vi "daq_FSM.vi"(8 "loop rate":u32=1000, 9 "commands":refnum<queue>, 11 "measurements":refnum<queue>) -> ()   [LabVIEW 2021, in "DAQ.lvlib"]
uses:
  DAQ.lvlib
  <vilib>/DAQmx/read.llb/DAQmx Read (Analog 1D DBL 1Chan NSamp).vi
  <vilib>/Analysis/baseanly.llb/Mean (DBL).vi
  <vilib>/DAQmx/create/channels.llb/DAQmx Create Channel (AI-Voltage-Basic).vi
  <vilib>/DAQmx/configure/timing.llb/DAQmx Timing (Sample Clock).vi
  <vilib>/DAQmx/miscellaneous.llb/DAQmx Fill In Error Info.vi
  <vilib>/Analysis/NI_AALBase.lvlib
panel:
  in  "STOP":bool
  out "Waveform Graph":dbl[](graph)
  in  "rate":dbl=1000.0 format="%0.2f"
  in  "samples per channel":i32=1000
  in  "physical channels":tag="Dev1/ai0"
  in  "error in":errorcluster
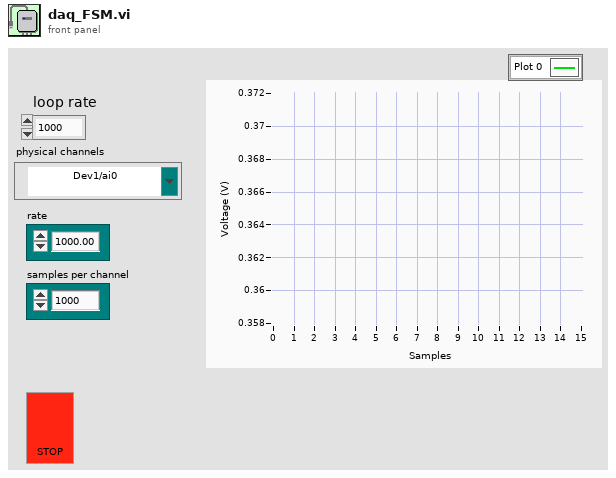
[diagram p1: front panel]
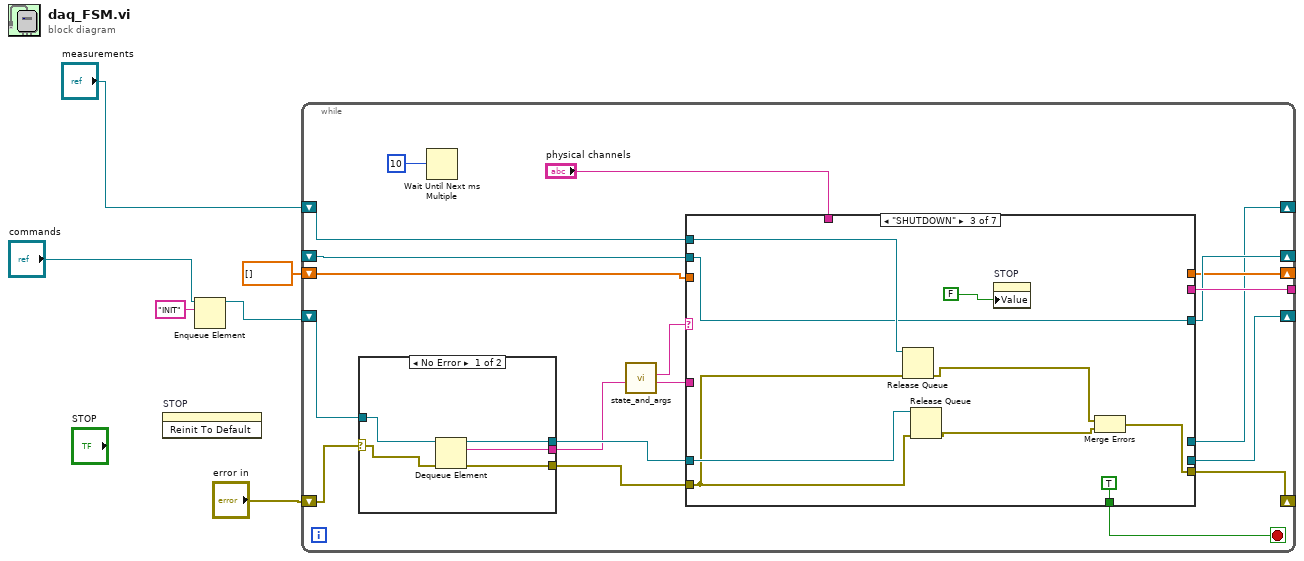
[diagram p0: block diagram]
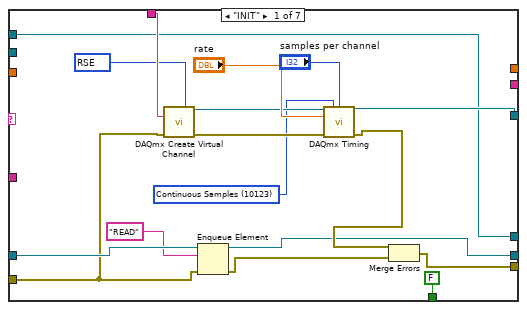
[diagram p2: hidden frame]
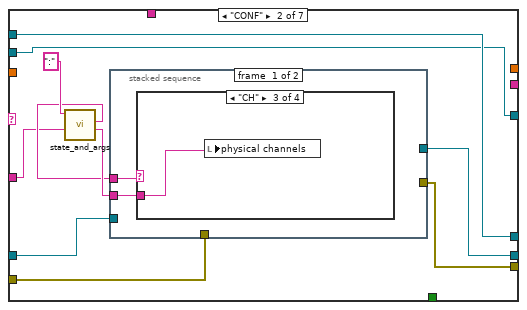
[diagram p3: hidden frame]
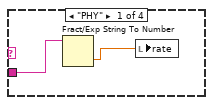
[diagram p4: hidden frame]
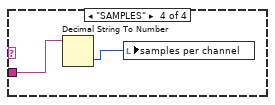
[diagram p6: hidden frame]
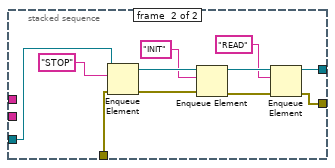
[diagram p7: hidden frame]
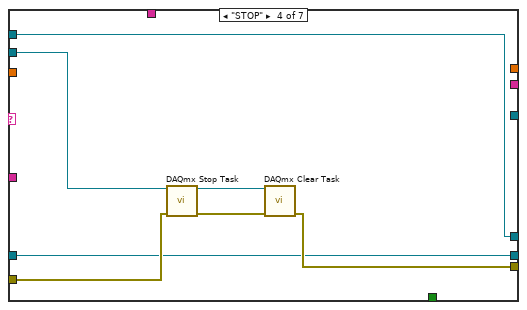
[diagram p8: hidden frame]
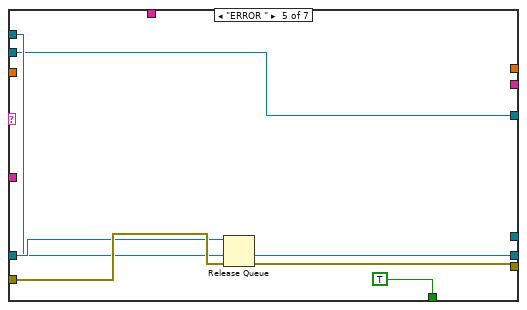
[diagram p9: hidden frame]
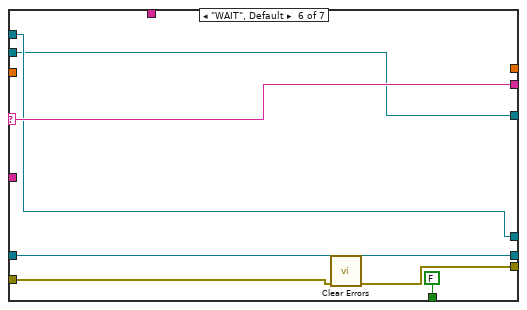
[diagram p10: hidden frame]
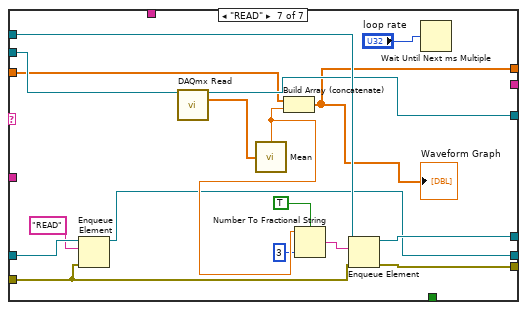
[diagram p11: hidden frame]
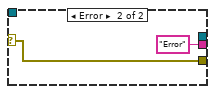
[diagram p12: hidden frame]
diagram:
  n1 = invoke on="STOP" class="Bool" method="Reinit To Default"() -> ()  [unwired: 3 in, 3 out]
  n2 = Enqueue Element(queue="commands", element="INIT") -> (queue out=w4:refnum<queue>)  [unwired: 2 in, 2 out]
  n3 = while {
    shift-right: [w15] -> _
    shift-left: "error in" -> [w25]
    tunnel: [w23] -> _
    shift-right: [w20] -> _
    shift-left: _ -> [w18]
    shift-right: [w10] -> _
    shift-left: dbl[] [] -> [w11]
    shift-right: [w8] -> _
    shift-left: w4 -> [w22]
    shift-right: [w9] -> _
    shift-left: "measurements" -> [w17]
    stop <- w14 stop-if-true
    n4 = case shown="No Error" w25 {
      selector: w25 -> [w119 w122]
      tunnel: [w121 "Error"] -> w13
      tunnel: w22 -> [w120 _]
      tunnel: [w118 w122] -> w21
      tunnel: [w117 _] -> w16
      frame No Error {
        n5 = Dequeue Element(queue=w120, error in (no error)=w119) -> (queue out=w117:refnum<queue>, element=w121:string, error out=w118:errorcluster)  [unwired: 1 in, 1 out]
      }
      frame Error {
      }
    }
    n6 = Wait Until Next ms Multiple(millisecond multiple=u32 10 ("millisecond timer value")) -> ()  [unwired: 1 out]
    n7 = call "state_and_args.vi"("String"=w13) -> ("Arguments"=w7:string, "State"=w12:string)  [unwired: 9 in]
    n8 = case shown="\"SHUTDOWN\"" w12 {
      selector: w12 -> [_ _ _ _ _ w99 _]
      tunnel: [_ _ _ _ _ w99 _] -> w23
      tunnel: w21 -> [w34 w49 w76 w85 w92 w97 w112]
      tunnel: [w37 w43 w71 _ w87 w93 w109] -> w20
      tunnel: "physical channels" -> [w42 _ _ _ _ _ _]
      tunnel: w18 -> [_ w43 w71 w86 w87 w93 w116]
      tunnel: w17 -> [w26 w44 w78 w81 w88 w95 w115]
      tunnel: w16 -> [w36 w51 w77 w80 w90 w94 w111]
      tunnel: [w26 w44 _ w81 _ w95 w113] -> w9
      tunnel: [w33 w50 w75 w82 w91 w96 w114] -> w15
      tunnel: [FALSE _ TRUE _ TRUE FALSE _] -> w14
      tunnel: w11 -> [_ _ _ _ _ _ w108]
      tunnel: [_ _ _ _ _ _ w102] -> w10
      tunnel: [w27 w45 _ w80 w88 w94 w100] -> w8
      tunnel: w7 -> [_ w46 _ _ _ _ _]
      frame "INIT" {
        w28 = 10083 items=["Default"=-1, "RSE"=10083, "NRSE"=10078, "Differential"=10106, "Pseudodifferential"=12529] ("input terminal configuration")
        w29 = 10123 items=["Finite Samples"=10178, "Continuous Samples"=10123, "Hardware Timed Single Point"=12522] ("sample mode")
        n9 = call-poly <vilib>:"DAQmx Create Virtual Channel.vi"("input terminal configuration"=w28, "physical channels"=w42, "error in"=w34) -> ("task out"=w39:refnum<k21>, "error out"=w38:errorcluster)  [unwired: 11 in]
        n10 = Enqueue Element(queue=w36, element="READ", error in (no error)=w34) -> (queue out=w27:refnum<queue>, error out=w32:errorcluster)  [unwired: 1 in, 1 out]
        n11 = call-poly <vilib>:"DAQmx Timing.vi"("task/channels in"=w39, "sample mode"=w29, "samples per channel"="samples per channel", "rate"="rate", "error in"=w38) -> ("task out"=w37:refnum<k21>, "error out"=w31:errorcluster)  [unwired: 9 in]
        n12 = Merge Errors(w31, w32) -> (w33:errorcluster)
      }
      frame "CONF" {
        n13 = call "state_and_args.vi"("String"=w46, "DELIMITER (:)"=":") -> ("Arguments"=w48:string, "State"=w47:string)  [unwired: 8 in]
        n14 = stacked-sequence {
          tunnel: w47 -> [w53 _]
          tunnel: [_ w63] -> w50
          tunnel: w48 -> [w54 _]
          tunnel: w51 -> [_ w62]
          tunnel: [_ w61] -> w45
          tunnel: w49 -> [_ w60]
          frame #0 {
            n15 = case shown="\"CH\"" w53 {
              tunnel: w54 -> [w55 _ w57 w58]
              frame "PHY" {
                n16 = Fract/Exp String To Number(string=w55) -> (number=w56:dbl)  [unwired: 3 in, 1 out]
                n17 = local write "rate"(w56) -> ()
              }
              frame Default {
              }
              frame "CH" {
                n18 = local write "physical channels"(w57) -> ()
              }
              frame "SAMPLES" {
                n19 = Decimal String To Number(string=w58) -> (number=w59:i32)  [unwired: 2 in, 1 out]
                n20 = local write "samples per channel"(w59) -> ()
              }
            }
          }
          frame #1 {
            n21 = Enqueue Element(queue=w62, element="STOP", error in (no error)=w60) -> (queue out=w70:refnum<queue>, error out=w69:errorcluster)  [unwired: 1 in, 1 out]
            n22 = Enqueue Element(queue=w70, element="INIT", error in (no error)=w69) -> (queue out=w66:refnum<queue>, error out=w65:errorcluster)  [unwired: 1 in, 1 out]
            n23 = Enqueue Element(queue=w66, element="READ", error in (no error)=w65) -> (queue out=w61:refnum<queue>, error out=w63:errorcluster)  [unwired: 1 in, 1 out]
          }
        }
      }
      frame "SHUTDOWN" {
        n24 = Release Queue(queue=w78, error in (no error)=w76) -> (error out=w74:errorcluster)  [unwired: 1 in, 2 out]
        n25 = Release Queue(queue=w77, error in (no error)=w76) -> (error out=w73:errorcluster)  [unwired: 1 in, 2 out]
        n26 = property on="STOP" class="Bool"("Value"=FALSE) -> ()  [unwired: 2 in, 2 out]
        n27 = Merge Errors(w74, w73) -> (w75:errorcluster)
      }
      frame "STOP" {
        n28 = call <vilib>:"DAQmx Stop Task.vi"("task/channels in"=w86, "error in"=w85) -> ("task out"=w84:refnum<k21>, "error out"=w83:errorcluster)  [unwired: 12 in]
        n29 = call <vilib>:"DAQmx Clear Task.vi"("task in"=w84, "error in"=w83) -> ("error out"=w82:errorcluster)  [unwired: 13 in]
      }
      frame "ERROR " {
        n30 = Release Queue(queue=w90, error in (no error)=w92) -> (error out=w91:errorcluster)  [unwired: 1 in, 2 out]
      }
      frame "WAIT", Default {
        n31 = call <vilib>:"Clear Errors.vi"("error in (no error)"=w97) -> ("error out"=w96:errorcluster)  [unwired: 5 in, 1 out]
      }
      frame "READ" {
        n32 = Enqueue Element(queue=w111, element="READ", error in (no error)=w112) -> (queue out=w100:refnum<queue>)  [unwired: 1 in, 2 out]
        n33 = call-poly <vilib>:"DAQmx Read.vi"("task/channels in"=w116) -> ("task out"=w109:refnum<k21>, "data"=w107:dbl[])  [unwired: 12 in, 1 out]
        n34 = call-poly <vilib>:"Mean.vi"("X"=w107) -> ("mean"=w103:dbl)  [unwired: 1 out]
        n35 = Build Array (concatenate)(w108, w103) -> (w102:dbl[])
        "Waveform Graph" <- w102
        n36 = Number To Fractional String(use system decimal point (T)=TRUE, number=w103, precision (6)=i16 3) -> (F-format string=w104:string)  [unwired: 1 in]
        n37 = Enqueue Element(queue=w115, element=w104, error in (no error)=w112) -> (queue out=w113:refnum<queue>, error out=w114:errorcluster)  [unwired: 1 in, 1 out]
        n38 = Wait Until Next ms Multiple(millisecond multiple="loop rate") -> ()  [unwired: 1 out]
      }
    }
  }
